vi "DATA_Extract.vi"(11 "Frame Queue":refnum<queue>) -> ()   [LabVIEW 2026]
uses:
  <vilib>/Platform/TimedLoop/XDataNode/wakeup.ctl
  <vilib>/Platform/TimedLoop/XDataNode/XDNodeRunTimeDep.lvlib
  <vilib>/Platform/TimedLoop/XDataNode/nitl_modes.ctl
  <vilib>/Platform/TimedLoop/XDataNode/timing_clust.ctl
  <vilib>/platform/TimedLoop/XDataNode/XDataNode.xnode
panel:
  in  "dataextraction":bool
  out "timed out? 3":bool
  out "concatenated string":string
  out "# elements in queue":i32
  out "abs(x) 4":i32
  out "element":u8[](array[numeric])
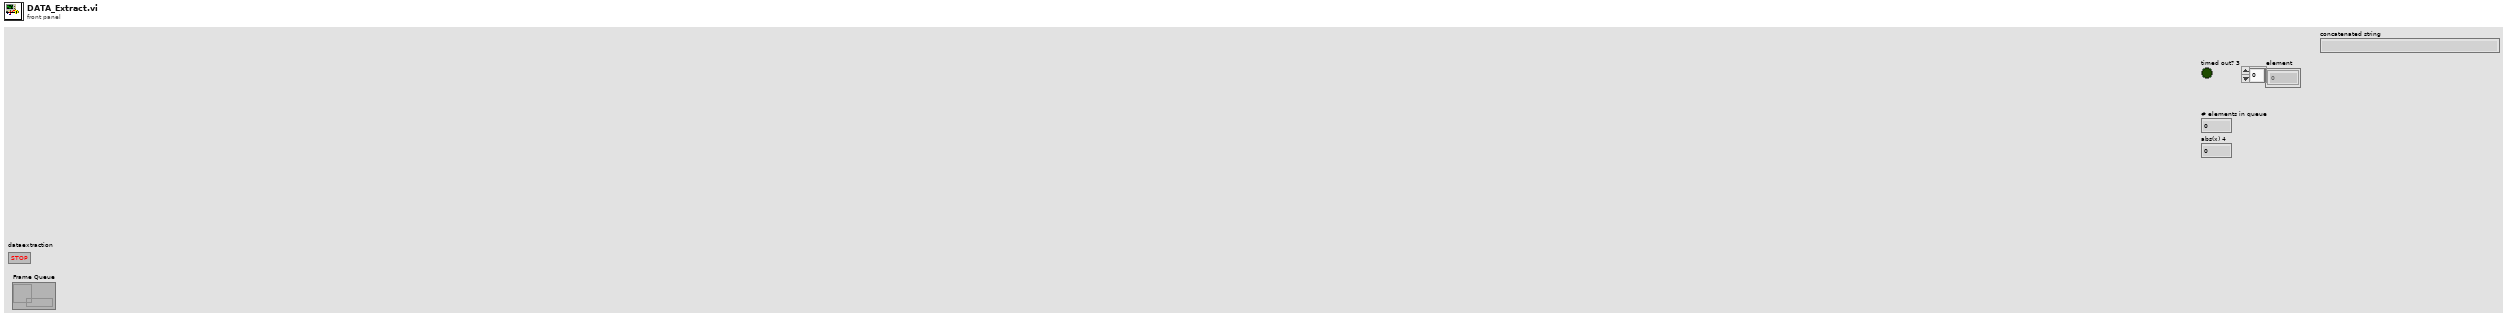
[diagram p1: front panel]
types:
  T1 = typedef "XDNodeRunTimeDep.lvlib/timing_clust.ctl" = cluster{"Expected End [f-1]":u64, "Actual End [f-1]":u64, "Finished Late? [f-1]":bool, "Expected End [i-1]":u64, "Actual End [i-1]":u64, "Finished Late? [i-1]":bool, "Expected Start [i]":u64, "Actual Start [i]":u64, "Expected Start [f]":u64, "Actual Start [f]":u64, "Source Name":string, "Structure Name":string, "Period":i64, "Deadline":i64, "Offset":i64, "Start":i64, "Priority":i32, "Timeout":i32, "Mode":T2, "Wakeup Reason":T3, "Error":errorcluster, "Source Type":string, "Secondary Source Type":string, "Global End Time":u64, "Global Start Time":u64, "Frame Duration":u64, "Iteration Duration":u64, "Assigned CPU":i32, "I/O Scan Engine Mode":u32}
  T2 = typedef "XDNodeRunTimeDep.lvlib/nitl_modes.ctl" = enum32{"No Change", "Process missed periods, maintain original phase", "Discard missed periods, maintain original phase", "Process missed periods, ignore original phase", "Discard missed periods, ignore original phase"}
  T3 = typedef "XDNodeRunTimeDep.lvlib/wakeup.ctl" = enum32{"Normal", "Aborted", "Asynchronous wakeup", "Timing source error", "Timed loop error", "Timeout"}
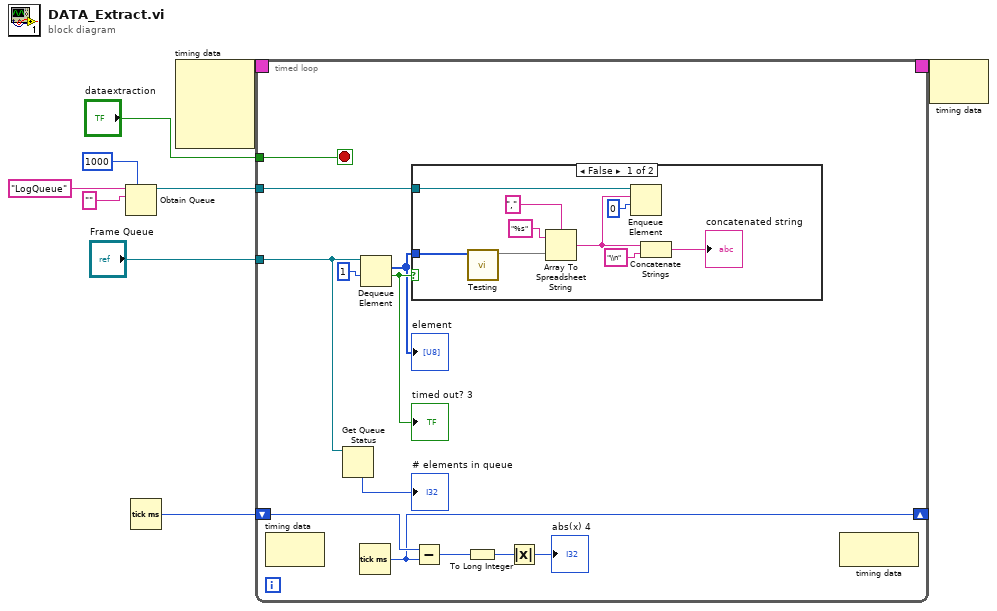
[diagram p0: block diagram]
diagram:
  n1 = Obtain Queue(max queue size (-1, unlimited)=1000, name (unnamed)="LogQueue", element data type="") -> (queue out=w1:refnum<queue>)  [unwired: 2 in, 2 out]
  n2 = Tick Count (ms)() -> (millisecond timer value=w7:u32)
  n3 = node-c288() -> (w9:T1)  [unwired: 4 in]
  n4 = timed-loop {
    timing: w9 -> [_]
    timing-out: [_] -> w8
    tunnel: "Frame Queue" -> [w14]
    shift-right: [w12] -> _
    shift-left: w7 -> [w13]
    tunnel: "dataextraction" -> [w11]
    tunnel: w1 -> [w10]
    stop <- w11 stop-if-true
    n5 = node-c288() -> ()  [unwired: 1 in, 1 out]
    n6 = Get Queue Status(queue=w14) -> (# elements in queue=→"# elements in queue":i32)  [unwired: 2 in, 7 out]
    n7 = Tick Count (ms)() -> (millisecond timer value=w12:u32)
    n8 = Dequeue Element(queue=w14, timeout in ms (-1)=1) -> (element=w19:u8[], timed out?=w20:bool)  [unwired: 1 in, 2 out]
    "timed out? 3" <- w20
    "element" <- w19
    n9 = case shown="False" w20 {
      tunnel: w19 -> [w30 _]
      tunnel: w10 -> [w25 _]
      frame False {
        n10 = call "Testing.vi"(11:w30) -> (3:w29)  [unwired: 10 in]
        n11 = Array To Spreadsheet String(delimiter (Tab)=",", array=w29, 3:"%s" ("format string")) -> (spreadsheet string=w23:string)
        n12 = Enqueue Element(queue=w25, element=w23, timeout in ms (-1)=0) -> ()  [unwired: 1 in, 3 out]
        n13 = Concatenate Strings(w23, "\\n" ("string")) -> (→"concatenated string":string)
      }
      frame True {
      }
    }
    n14 = Subtract(x=w13, y=w12) -> (x-y=w17:u32)
    n15 = To Long Integer(number=w17) -> (32bit integer=w16:i32)
    n16 = Absolute Value(x=w16) -> (abs(x)=→"abs(x) 4":i32)
    n17 = node-c288() -> ()  [unwired: 1 in, 1 out]
  }
  n18 = node-c288(w8) -> ()  [unwired: 1 out]
